vi "UsrProfiles-Delete profiles of single user.vi"(8 "error in":errorcluster, 11 "Name of user to remove":string) -> (0 "error out":errorcluster)   [LabVIEW 2013]
uses:
  Typedefs/Which path.ctl
  Globals/gl_UsrProfiles globals.vi
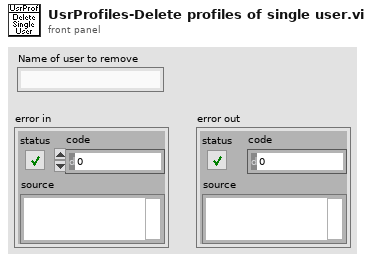
[diagram p1: front panel]
types:
  T1 = typedef "Which path.ctl" = enum16{"Configuration Files", "Calibration Files", "Images", "Setup.ini", "Loaded User profile.ini", "User's-Previous session.ini", "New user profile.ini", "Selected User profile.ini", "User profiles folder", "Power meter scaling.txt", "FOV Cal.ini"}
  T2 = typedef "User login window refs.ctl" = cluster{"User profiles window ref":refnum<k9>, "Users listbox":refnum<vi>, "Profiles listbox":refnum<vi>, "Last used":refnum<vi>}
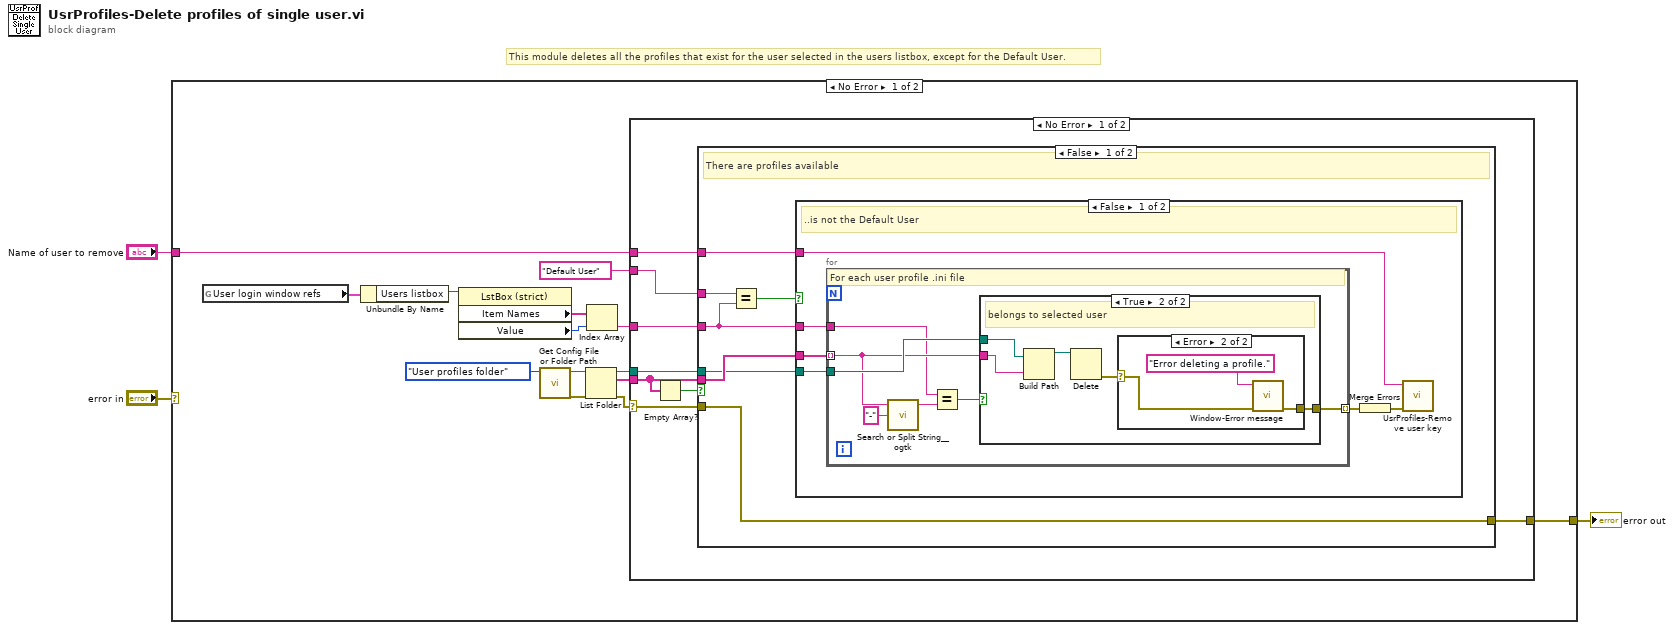
[diagram p0: block diagram]
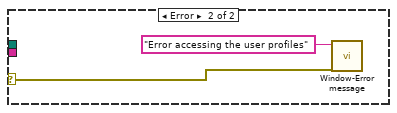
[diagram p6: hidden frame]
diagram:
  # "This module deletes all the profiles that exist for the user selected in the users listbox, except for the Default User."
  n1 = case shown="No Error" "error in" {
    selector: "error in" -> [_ w57]
    tunnel: [w12 w57] -> w3
    tunnel: "Name of user to remove" -> [w4 _]
    frame No Error {
      n2 = global read "gl_UsrProfiles globals.vi" "User login window refs"() -> (w11:T2)
      n3 = Unbundle By Name(w11) -> ("Users listbox"=w10:refnum<vi>)
      n4 = property class="LstBox (strict)"(reference=w10) -> ("Item Names"=w9:string[], "Value"=w8:i32)  [unwired: 1 in, 2 out]
      n5 = call "Get Config File or Folder Path.vi"("Which file or folder?"=Which_path."User profiles folder") -> ("Error Out"=w15:errorcluster, "File Path"=w16:path)  [unwired: 8 in, 1 out]
      n6 = List Folder(path=w16, error in=w15) -> (path out=w5:path, filenames=w13:string[], error out=w14:errorcluster)  [unwired: 2 in, 1 out]
      n7 = Index Array(array=w9, index=w8) -> (element=w7:string)
      n8 = case shown="No Error" w14 {
        selector: w14 -> [w24 w56]
        tunnel: w13 -> [w22 _]
        tunnel: [w23 _] -> w12
        tunnel: w7 -> [w21 _]
        tunnel: "Default User" -> [w20 _]
        tunnel: w5 -> [w19 _]
        tunnel: w4 -> [w18 _]
        frame No Error {
          n9 = Empty Array?(array=w22) -> (empty?=w25:bool)
          n10 = case shown="False" w25 {
            tunnel: w22 -> [w32 _]
            tunnel: w24 -> [w31 w54]
            tunnel: [w31 w54] -> w23
            tunnel: w21 -> [w30 _]
            tunnel: w20 -> [w29 _]
            tunnel: w19 -> [w27 _]
            tunnel: w18 -> [w26 _]
            frame False {
              # "There are profiles available"
              n11 = Equal?(x=w29, y=w30) -> (x = y?=w28:bool)
              n12 = case shown="False" w28 {
                tunnel: w32 -> [w38 _]
                tunnel: w30 -> [w37 _]
                tunnel: w27 -> [w36 _]
                tunnel: w26 -> [w33 _]
                frame False {
                  # "..is not the Default User"
                  n13 = for {
                    tunnel: w38 -> [w42] mode=indexing
                    tunnel: w37 -> [w40]
                    tunnel: w36 -> [w45]
                    tunnel: [w44] -> w35 mode=indexing
                    # "For each user profile .ini file"
                    n14 = call "Search or Split String__ogtk.vi"("search string/char (-)"="-", "string"=w42) -> ("substring before match"=w41:string)  [unwired: 1 in, 2 out]
                    n15 = Equal?(x=w40, y=w41) -> (x = y?=w39:bool)
                    n16 = case shown="True" w39 {
                      tunnel: w42 -> [_ w49]
                      tunnel: w45 -> [_ w50]
                      tunnel: [_ w46] -> w44
                      frame False {
                      }
                      frame True {
                        # "belongs to selected user"
                        n17 = Build Path(base path=w50, name or relative path=w49) -> (appended path=w48:path)
                        n18 = Delete(path (use dialog)=w48) -> (error out=w47:errorcluster)  [unwired: 4 in, 2 out]
                        n19 = case shown="Error" w47 {
                          selector: w47 -> [_ w53]
                          tunnel: [_ w51] -> w46
                          frame No Error {
                          }
                          frame Error {
                            n20 = call "Window-Error message.vi"("error in (no error)"=w53, "Message"="Error deleting a profile.") -> ("Error Out (no error)"=w51:errorcluster)  [unwired: 9 in]
                          }
                        }
                      }
                    }
                  }
                  n21 = Merge Errors(w35) -> (w34:errorcluster)
                  n22 = call "UsrProfiles-Remove user key.vi"("error in (no error)"=w34, "Name of user to remove"=w33) -> ()  [unwired: 10 in]
                }
                frame True {
                  # "Default User"
                }
              }
            }
            frame True {
              # "No profiles available. Even the default profile is missing."
            }
          }
        }
        frame Error {
          n23 = call "Window-Error message.vi"("error in (no error)"=w56, "Message"="Error accessing the user profiles") -> ()  [unwired: 9 in, 1 out]
        }
      }
    }
    frame Error {
    }
  }
  "error out" <- w3
